vi "Signal-error.vi"(8 "error in (no error)":errorcluster, 11 "Data ref. in":refnum<data-value>) -> (0 "error out":errorcluster, 3 "Data ref.":refnum<data-value>)   [LabVIEW 2013, in "CameraVision.lvlib" / "CV-Main.lvclass"]
uses:
  CV-Main.lvclass
  CV-Main.lvclass/CV-Main.ctl
  Errors/CV-Errors.lvclass/CV-Errors.ctl
  Read Errors.vi
  Errors/Read Error event.vi
  Errors/CV-Errors.lvclass
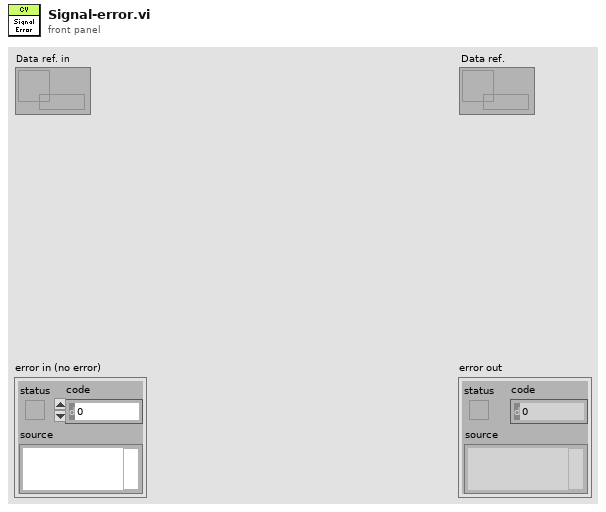
[diagram p1: front panel]
types:
  T1 = typedef "CameraVision.lvlib/CV-Errors.lvclass/Object-reference.ctl" = refnum<data-value>
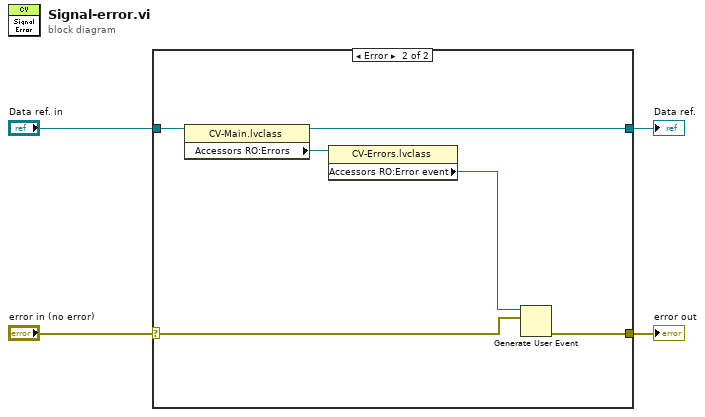
[diagram p0: block diagram]
diagram:
  n1 = case shown="Error" "error in (no error)" {
    selector: "error in (no error)" -> [w5 w12]
    tunnel: [w5 w11] -> w3
    tunnel: [w6 w9] -> w1
    tunnel: "Data ref. in" -> [w6 w10]
    frame No Error {
    }
    frame Error {
      n2 = property class="CV-Main.lvclass"(reference=w10) -> (reference out=w9:refnum<data-value>, "Accessors RO:Errors"=w8:T1)  [unwired: 1 in, 1 out]
      n3 = property class="CV-Errors.lvclass"(reference=w8) -> ("Accessors RO:Error event"=w7:refnum<user-event>)  [unwired: 1 in, 2 out]
      n4 = Generate User Event(user event=w7, event data cluster=w12) -> (error out=w11:errorcluster)  [unwired: 2 in, 1 out]
    }
  }
  "error out" <- w3
  "Data ref." <- w1
